vi "SendMessage.vi"(8 "error in (no error)":errorcluster, 9 "Message Data":variant, 10 "Message":string="Exit", 11 "JQMHModule in":refnum<class "JQMHModule.lvclass">) -> (0 "error out":errorcluster, 3 "JQMHModule out":refnum<class "JQMHModule.lvclass">)   [LabVIEW 2024, in "JQMHModule.lvclass"]
uses:
  JQMHModule.lvclass
  JQMHModule.lvclass/JQMHModule.ctl
  Message Queue_class/JQMH_Message Queue.lvclass/JQMH_Message Queue.ctl
  Message Queue_class/Delacor_lib_QMH_Enqueue Message (Single).vi
  Message Queue_class/JQMH_Message Queue.lvclass
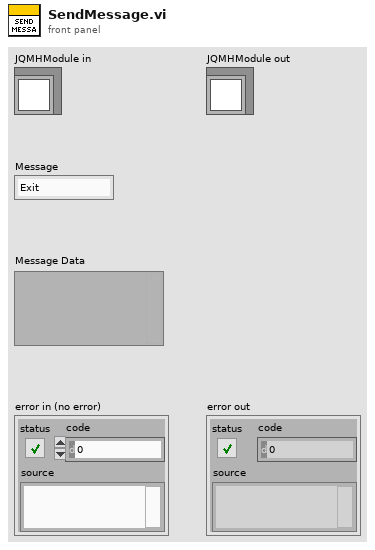
[diagram p1: front panel]
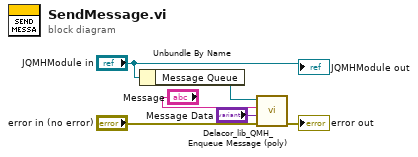
[diagram p0: block diagram]
diagram:
  n1 = Unbundle By Name("JQMHModule in") -> ("Message Queue"=w3:refnum<class "QMH_Message Queue.lvclass">)
  n2 = call-poly "Delacor_lib_QMH_Enqueue Message (poly).vi"("error in"="error in (no error)", "Message Data"="Message Data", "Message"="Message", "Message Queue in"=w3) -> ("error out"=→"error out":errorcluster)  [unwired: 6 in, 1 out]
  "JQMHModule out" <- "JQMHModule in"
